vi "Write to File.vi"(8 "error in":errorcluster, 11 "File Actor in":refnum<class "File Actor.lvclass">) -> (0 "error out":errorcluster, 3 "File Actor out":refnum<class "File Actor.lvclass">)   [LabVIEW 2014, in "File Library.lvlib" / "File Actor.lvclass"]
doc: "This is the routine that actually performs the file writing. It should reside in the non-message handling portion of the Actor Core. It may be overriden to handle\n\n1. different file formats\n2. different data formats."
uses:
  File Actor.lvclass
  <vilib>/ActorFramework/Actor/Actor.lvclass/Actor.ctl
  File Actor.lvclass/File Actor.ctl
  Messages/Abstract/Saving File Message/Saving File Message.lvclass
  Messages/Abstract/Saving File Message/Saving File Message.lvclass/Saving File Message.ctl
  <vilib>/ActorFramework/Message Enqueuer/Message Enqueuer.lvclass/Message Enqueuer.ctl
  <vilib>/ActorFramework/Message Priority Queue/Priority Enqueue.vi
  reusable/Data/Data.lvclass
  <vilib>/ActorFramework/Actor/Actor.lvclass
  <vilib>/ActorFramework/Message Enqueuer/Message Enqueuer.lvclass
  reusable/Session APIs/Session Log/System Log.lvclass
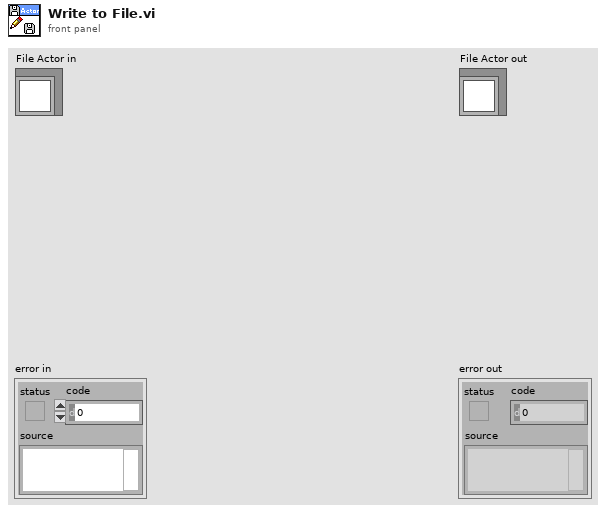
[diagram p1: front panel]
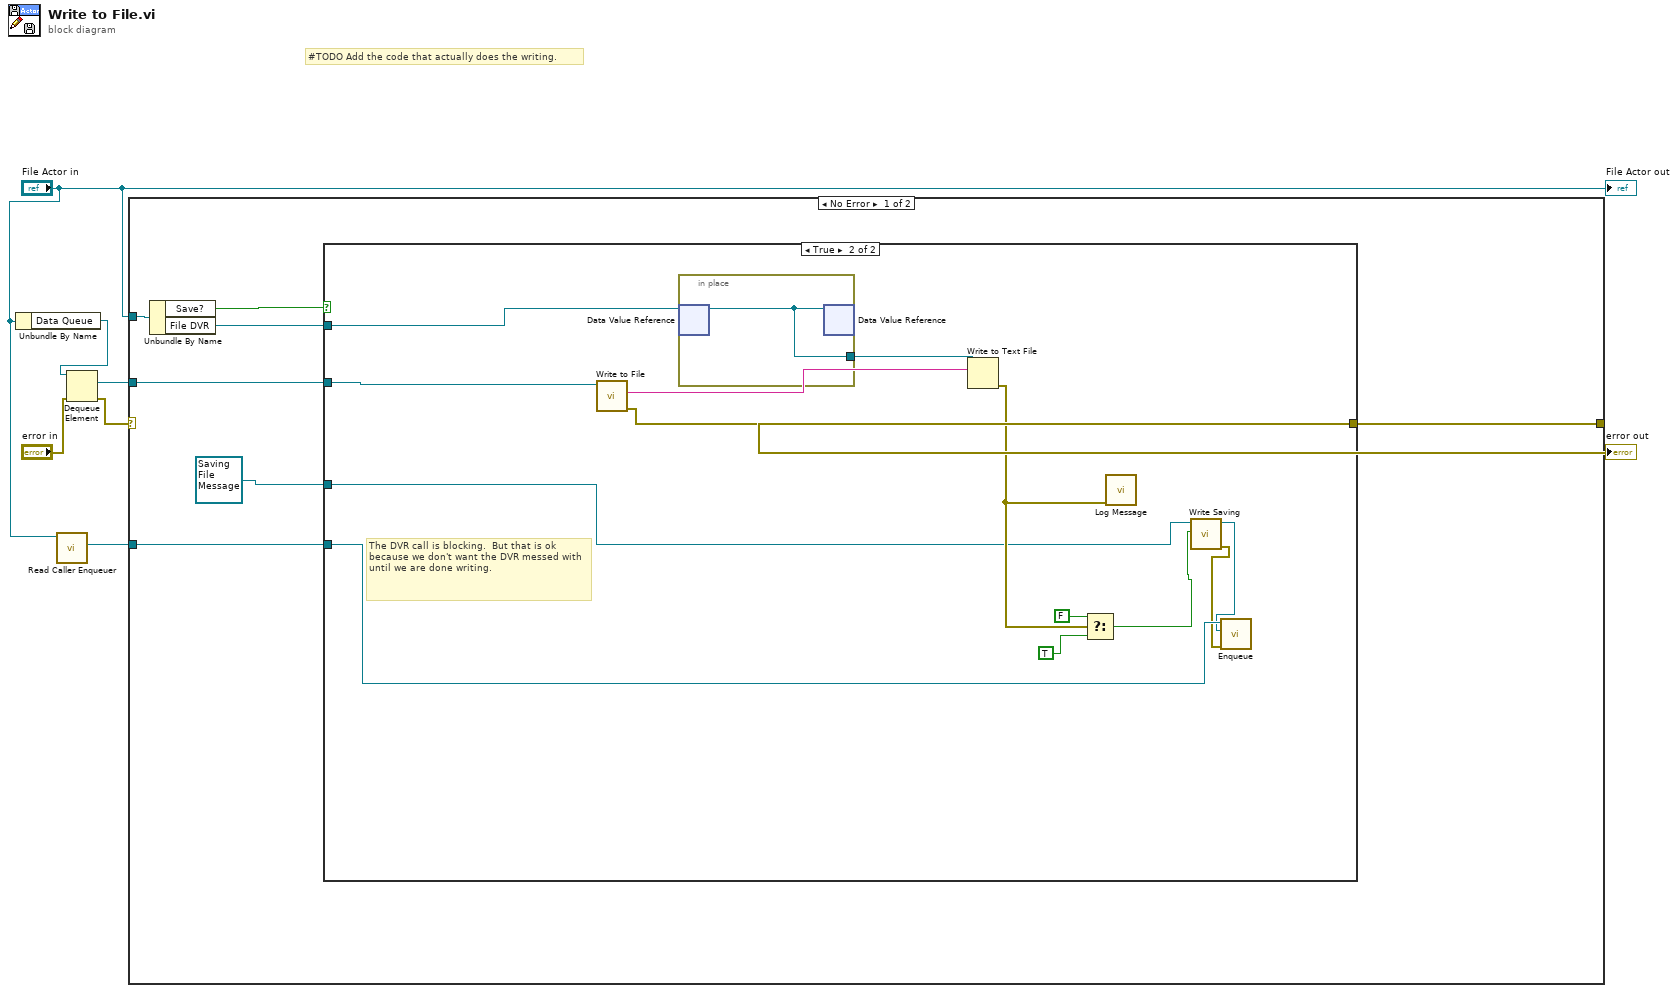
[diagram p0: block diagram]
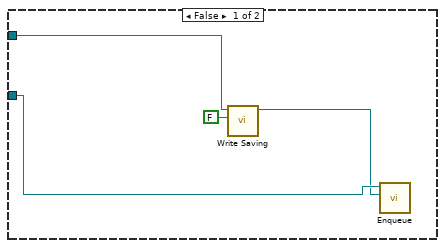
[diagram p2: hidden frame]
diagram:
  # "#TODO Add the code that actually does the writing."
  n1 = Unbundle By Name("File Actor in") -> ("Data Queue"=w7:refnum<queue>)
  n2 = call <vilib>:"Read Caller Enqueuer.vi"("Actor"="File Actor in") -> ("Caller Enqueuer"=w1:refnum<class "Message Enqueuer.lvclass">)  [unwired: 10 in]
  n3 = Dequeue Element(queue=w7, error in (no error)="error in") -> (element=w6:refnum<class "Data.lvclass">, error out=w4:errorcluster)  [unwired: 1 in, 2 out]
  n4 = case shown="No Error" w4 {
    selector: w4 -> [_ w33]
    tunnel: "File Actor in" -> [w12 _]
    tunnel: w6 -> [w14 _]
    tunnel: [w13 w33] -> w3
    tunnel: w1 -> [w9 _]
    frame No Error {
      n5 = Unbundle By Name(w12) -> ("Save?"=w10:bool, "File DVR"=w11:refnum<data-value>)
      n6 = case shown="True" w10 {
        tunnel: w14 -> [_ w31]
        tunnel: [_ w30] -> w13
        tunnel: w11 -> [_ w29]
        tunnel: refnum<class "Saving File Message.lvclass"> refnum ("File Library.lvlib:Saving Main File MSG") -> [w17 w22]
        tunnel: w9 -> [w18 w23]
        frame False {
          n7 = call "Write Saving.vi"("Saving"=FALSE, "Saving File Message in"=w17) -> ("Saving File Message out"=w15:refnum<class "Saving File Message.lvclass">)  [unwired: 8 in, 1 out]
          n8 = call <vilib>:"Enqueue.vi"("Message"=w15, "Message Enqueuer in"=w18) -> ()  [unwired: 8 in, 2 out]
        }
        frame True {
          # "The DVR call is blocking.  But that is ok because we don't want the DVR messed with until we are done writing."
          n9 = call-dynamic "Write to File.vi"("Data in"=w31) -> ("error out"=w30:errorcluster, "Serialized Data Out"=w27:string)  [unwired: 8 in, 1 out]
          n10 = in-place {
            in-place-border: [w32] -> w28
            n11 = in-place-dvr #1(w29) -> (w32:refnum<file>)  [unwired: 1 out]
            n12 = in-place-dvr #1(w32) -> ()  [unwired: 2 out]
          }
          n13 = Write to Text File(file (use dialog)=w28, text=w27) -> (error out=w26:errorcluster)  [unwired: 2 in, 2 out]
          n14 = Select(t=FALSE, s=w26, f=TRUE) -> (s? t:f=w21:bool)
          n15 = call "Log Message.vi"("error in"=w26) -> ()  [unwired: 9 in, 2 out]
          n16 = call "Write Saving.vi"("Saving"=w21, "Saving File Message in"=w22) -> ("error out"=w19:errorcluster, "Saving File Message out"=w20:refnum<class "Saving File Message.lvclass">)  [unwired: 8 in]
          n17 = call <vilib>:"Enqueue.vi"("error in (no error)"=w19, "Message"=w20, "Message Enqueuer in"=w23) -> ()  [unwired: 7 in, 2 out]
        }
      }
    }
    frame Error {
    }
  }
  "error out" <- w3
  "File Actor out" <- "File Actor in"
